vi "Print.vi"(6 "Byte Count (1024)":u32=1024, 8 "error in (no error)":errorcluster, 9 "Input":string, 11 "VISA resource name":refnum<visa-resource-name>) -> (0 "error out":errorcluster, 1 "Output":string, 3 "VISA resource name out":refnum<visa-resource-name>, 4 "Command String":string)   [LabVIEW 2018, in "Keithley 3706.lvlib"]
uses:
  <instrlib>/Keithley 3706/Keithley 3706.lvlib
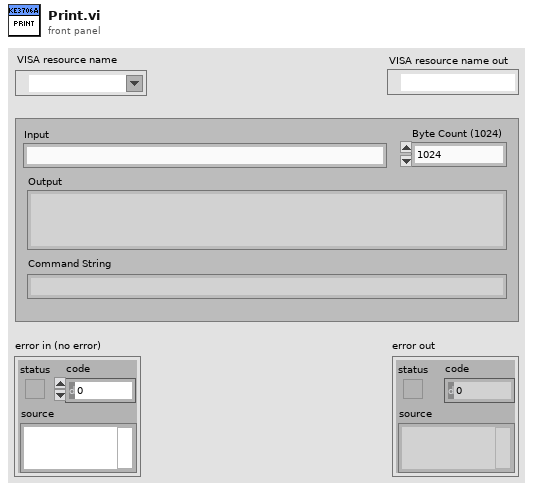
[diagram p1: front panel]
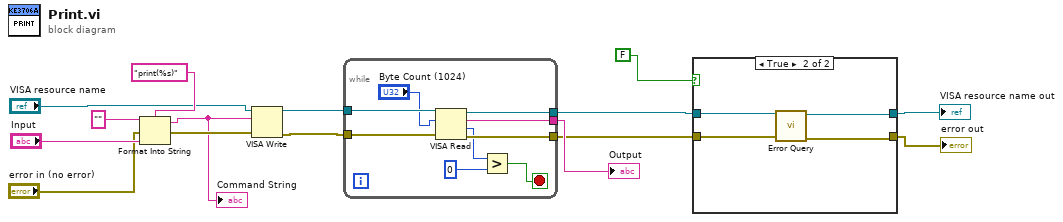
[diagram p0: block diagram]
diagram:
  n1 = Format Into String(format string="print(%s)", initial string="", error in="error in (no error)", "Input") -> (resulting string=w10:string, error out=w11:errorcluster)
  "Command String" <- w10
  n2 = VISA Write(VISA resource name="VISA resource name", write buffer=w10, error in (no error)=w11) -> (VISA resource name out=w8:refnum<visa-resource-name>, error out=w7:errorcluster)  [unwired: 1 out]
  n3 = while {
    tunnel: w8 -> [w24]
    tunnel: w7 -> [w23]
    tunnel: [w21] -> w5
    tunnel: [w20] -> w4
    tunnel: [w19] -> w6
    stop <- w16 stop-if-true
    n4 = VISA Read(VISA resource name=w24, byte count="Byte Count (1024)", error in (no error)=w23) -> (VISA resource name out=w21:refnum<visa-resource-name>, read buffer=w19:string, return count=w18:u32, error out=w20:errorcluster)
    n5 = Greater?(x=w18, y=0) -> (0:w16:bool)
  }
  "Output" <- w6
  n6 = case shown="True" FALSE {
    tunnel: w5 -> [w26 w30]
    tunnel: w4 -> [w25 w29]
    tunnel: [w26 w28] -> w2
    tunnel: [w25 w27] -> w1
    frame False {
    }
    frame True {
      n7 = call <instrlib>:"Error Query.vi"("error in (no error)"=w29, "VISA resource name"=w30) -> ("error out"=w27:errorcluster, "VISA resource name output"=w28:refnum<visa-resource-name>)  [unwired: 6 in, 2 out]
    }
  }
  "VISA resource name out" <- w2
  "error out" <- w1
